vi "Protection Settings.vi"(6 "Action":enum8{"Get", "Set"}(ring), 8 "error in":errorcluster, 10 "Selected Channels":T1 {"Input Channels"."Node Ref" format="%.0x"}, 11 "Parent Ref":T3=18446744073709551615 format="%.0x") -> (0 "error out":errorcluster, 2 "Selected Channels":T1 {"Input Channels"."Node Ref" format="%.0x"}, 3 "Parent Ref Out":T3=18446744073709551615 format="%.0x")   [LabVIEW 2015, in "Protection and Counter Support System Explorer.lvlib"]
uses:
  Protection and Counter Support System Explorer.lvlib
  <vilib>/NI Veristand/Custom Device API/Custom Device Item Ref.ctl
  Types/Protection Signal Settings.ctl
  Types/Protection Signal Linked Channel.ctl
  Shared/Types/Protection Type.ctl
  Shared/Properties Lookup.vi
  <vilib>/NI Veristand/Custom Device API/Set Item Property (Dependent Node Pointer).vi
  <vilib>/NI Veristand/Custom Device API/Set Item Property (String Array).vi
  <vilib>/NI Veristand/Custom Device API/Set Item Property (U32).vi
  <vilib>/NI Veristand/Custom Device API/Get Item Property (String Array).vi
  <vilib>/NI Veristand/Custom Device API/Get Item Property (Dependent Node Pointer).vi
  <vilib>/NI Veristand/Custom Device API/Get Item Property (U32).vi
  <vilib>/NI VeriStand/Custom Device API/Custom Device API.lvlib
  Shared/Protection and Counter Support Shared.lvlib
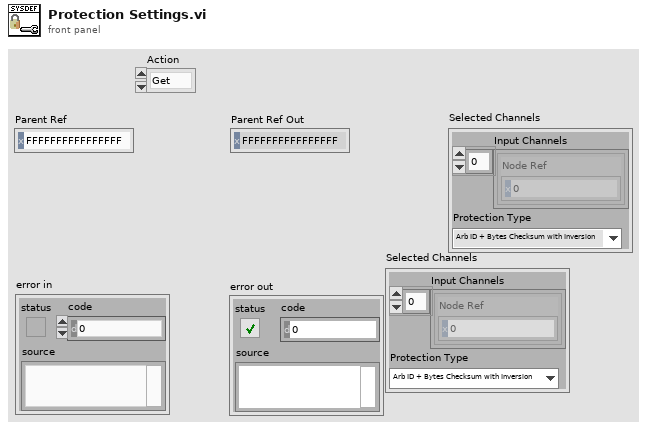
[diagram p1: front panel]
types:
  T1 = typedef "Protection and Counter Support System Explorer.lvlib/Protection Signal Settings.ctl" = cluster{"Input Channels":T2[], "Protection Type":T4}
  T2 = typedef "Protection and Counter Support System Explorer.lvlib/Protection Signal Linked Channel.ctl" = cluster{"Node Ref":T3}
  T3 = typedef "Custom Device API.lvlib/Custom Device Item Ref.ctl" = u64
  T4 = typedef "Protection and Counter Support Shared.lvlib/Protection Type.ctl" = enum16{"Arb ID + Bytes Checksum with Inversion", "Arb ID + Bytes CRC with Inversion (Little Endian Only)", "Reversed Raw Signal Checksum with Inversion"}
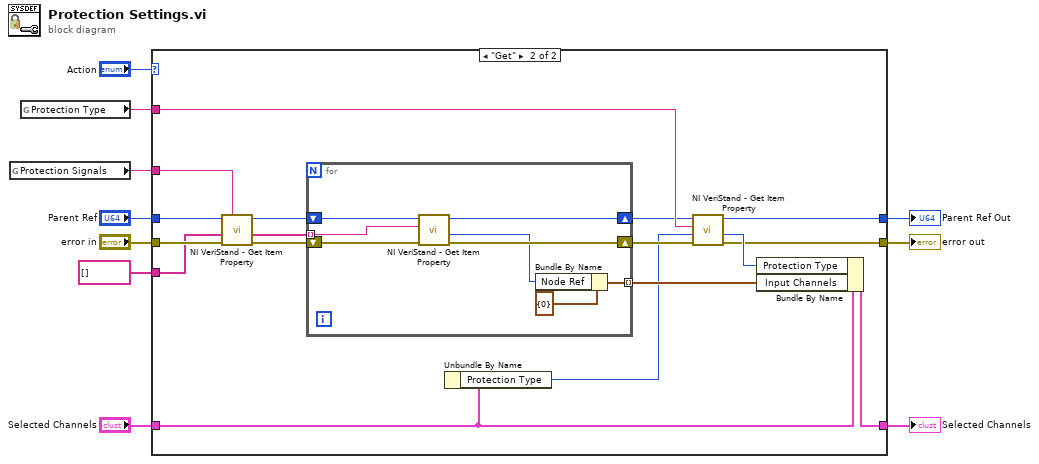
[diagram p0: block diagram]
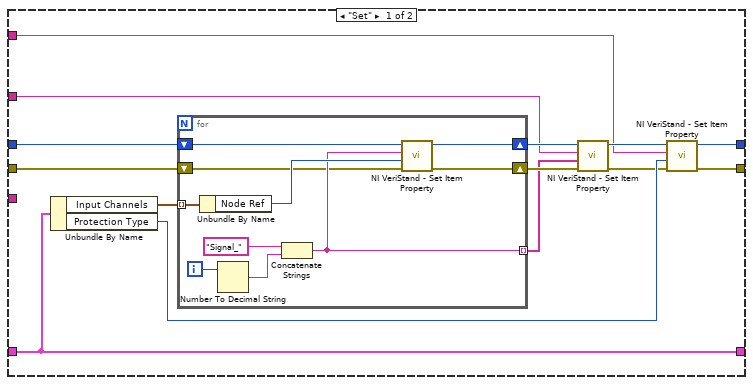
[diagram p2: hidden frame]
diagram:
  n1 = global read "Properties Lookup.vi" "Protection Signals"() -> (w1:string)
  n2 = global read "Properties Lookup.vi" "Protection Type"() -> (w2:string)
  n3 = case shown="\"Get\"" "Action" {
    tunnel: "error in" -> [w17 w51]
    tunnel: "Parent Ref" -> [w16 w50]
    tunnel: w1 -> [w15 w49]
    tunnel: string[] [] -> [_ w48]
    tunnel: w2 -> [w14 w45]
    tunnel: "Selected Channels" -> [w11 w36]
    tunnel: [w11 w43] -> w7
    tunnel: [w13 w39] -> w6
    tunnel: [w12 w37] -> w5
    frame "Set" {
      n4 = Unbundle By Name(w11) -> ("Input Channels"=w24:T2[], "Protection Type"=w19:T4)
      n5 = for {
        tunnel: w24 -> [w31] mode=indexing
        tunnel: [w29] -> w21 mode=indexing
        shift-right: [w27] -> w23
        shift-left: w17 -> [w28]
        shift-right: [w25] -> w22
        shift-left: w16 -> [w26]
        i -> [w33]
        n6 = Unbundle By Name(w31) -> ("Node Ref"=w30:T3)
        n7 = Number To Decimal String(number=w33) -> (decimal integer string=w32:string)  [unwired: 1 in]
        n8 = Concatenate Strings("Signal_" ("string"), w32) -> (w29:string)
        n9 = call-poly <vilib>:"NI VeriStand - Set Item Property.vi"("error in (no error)"=w28, "Dependent Node Ref"=w30, "Property Name"=w29, "Item Ref in"=w26) -> ("error out"=w27:errorcluster, "Item Ref out"=w25:T3)  [unwired: 5 in, 1 out]
      }
      n10 = call-poly <vilib>:"NI VeriStand - Set Item Property.vi"("error in (no error)"=w23, "Value"=w21, "Property Name"=w15, "Item Ref in"=w22) -> ("error out"=w18:errorcluster, "Item Ref out"=w20:T3)  [unwired: 5 in, 1 out]
      n11 = call-poly <vilib>:"NI VeriStand - Set Item Property.vi"("error in (no error)"=w18, "Value"=w19, "Property Name"=w14, "Item Ref in"=w20) -> ("error out"=w13:errorcluster, "Item Ref out"=w12:T3)  [unwired: 5 in, 1 out]
    }
    frame "Get" {
      n12 = call-poly <vilib>:"NI VeriStand - Get Item Property.vi"("error in (no error)"=w51, "Default Value"=w48, "Property Name"=w49, "Item Ref in"=w50) -> ("error out"=w47:errorcluster, "Value"=w42:string[], "Item Ref out"=w46:T3)  [unwired: 4 in, 1 out]
      n13 = for {
        shift-right: [w57] -> w38
        shift-left: w46 -> [w58]
        tunnel: w42 -> [w56] mode=indexing
        shift-right: [w55] -> w41
        shift-left: w47 -> [w59]
        tunnel: [w52] -> w40 mode=indexing
        n14 = call-poly <vilib>:"NI VeriStand - Get Item Property.vi"("error in (no error)"=w59, "Property Name"=w56, "Item Ref in"=w58) -> ("error out"=w55:errorcluster, "Dependent Node Ref"=w53:T3, "Item Ref out"=w57:T3)  [unwired: 5 in, 1 out]
        n15 = Bundle By Name(cluster=T2 {"Node Ref"=0} ("MonitoredChannelSettings"), "Node Ref"=w53) -> (w52:T2)
      }
      n16 = Unbundle By Name(w36) -> ("Protection Type"=w35:T4)
      n17 = call-poly <vilib>:"NI VeriStand - Get Item Property.vi"("error in (no error)"=w41, "Default Value"=w35, "Property Name"=w45, "Item Ref in"=w38) -> ("error out"=w39:errorcluster, "Value"=w44:u32, "Item Ref out"=w37:T3)  [unwired: 4 in, 1 out]
      n18 = Bundle By Name(cluster=w36, "Protection Type"=w44, "Input Channels"=w40) -> (w43:T1)
    }
  }
  "error out" <- w6
  "Parent Ref Out" <- w5
  "Selected Channels" <- w7
